vi "Global 2.vi"() -> ()   [LabVIEW 2019]
panel:
  out "CAMARELO":dbl
  out "CVERDE":dbl
  out "CVERMELHO":dbl
  out "CAZUL":dbl
  out "AMARELO":dbl
  out "VERDE":dbl
  out "VERMELHO":dbl
  out "AZUL":dbl
  out "botão":bool
  out "controle":dbl
  in  "COR":string
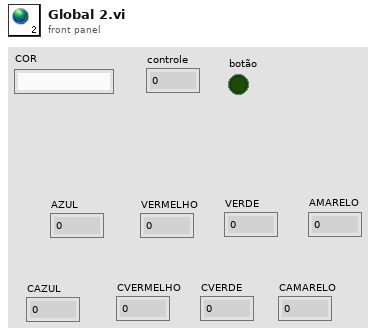
[diagram p1: front panel]
diagram:
